vi "Initialize.vi"(0 "VISA resource name":refnum<visa-resource-name>, 7 "Serial Configuration":T1={"Baud Rate (19200)"=19200, "Parity (0: None)"=0, "Break Length (0)"=20} {"Break Length (0)" items=["0"=10, "1.5"=15, "2.0"=20]; "Parity (0: None)" items=["None", "Odd", "Even"]; "Baud Rate (19200)" items=["1200"=1200, "2400"=2400, "4800"=4800, "9600"=9600, "19200"=19200]}, 11 "error in (no error)":errorcluster) -> (4 "VISA resource name out":refnum<visa-resource-name>, 15 "error out":errorcluster {"code" format="%x"})   [LabVIEW 2010, in "Eurotherm 32xx Series.lvlib"]
doc: "This VI passes the addressing information in the instrument decriptor to the Instr Open VI and returns the instrument ID. You must run this VI before using any of the instrument driver VIs for this instrument.\n\nNotes:\n\n(1) This instrument driver supports serial communication. If problems are encountered when using serial communication, it is recommended to try using baud rates less than 19,200 and hardware handshaking. \n\n(2) If you do wish to use the serial interface, set the serial settings on the instrument to be the same as the serial settings on the block diagram and in Measurement & Automation Explorer."
uses:
  <instrlib>/Eurotherm 32xx Series/Eurotherm 32xx Series.lvlib
panel:
  # "(c) 2010 <Invensys Eurotherm>.  ALL RIGHTS RESERVED."
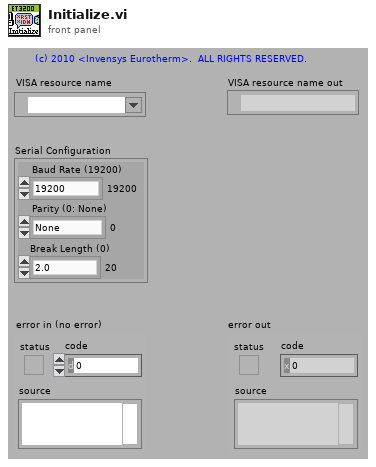
[diagram p1: front panel]
types:
  T1 = cluster{"Baud Rate (19200)":u32, "Parity (0: None)":u16, "Break Length (0)":u16}
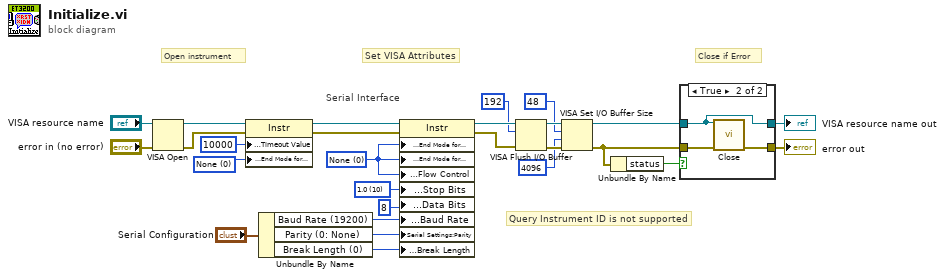
[diagram p0: block diagram]
diagram:
  w5 = u16 10 items=["1.0"=10, "1.5"=15, "2.0"=20] ("Serial Settings:Serial Stop Bits")
  w6 = u16 0 items=["None", "LastBit", "TermChar"] ("Serial Settings:Serial End Mode for Reads")
  w17 = u16 0 items=["None", "LastBit", "TermChar"] ("Serial Settings:Serial End Mode for Reads")
  # "Serial Interface"
  # "Set VISA Attributes"
  # "Close if Error"
  # "Query Instrument ID is not supported"
  # "Open instrument"
  n1 = VISA Open(error in (no error)="error in (no error)", VISA resource name="VISA resource name") -> (VISA resource name=w16:refnum<visa-resource-name>, error out=w15:errorcluster)  [unwired: 3 in]
  n2 = property class="Instr"(reference=w16, error in=w15, "General Settings:Timeout Value"=u32 10000, "Serial Settings:End Mode for Reads"=w17) -> (reference out=w20:refnum<visa-resource-name>, error out=w19:errorcluster)
  n3 = Unbundle By Name("Serial Configuration") -> ("Baud Rate (19200)"=w3:u32, "Parity (0: None)"=w2:u16, "Break Length (0)"=w1:u16)
  n4 = property class="Instr"(reference=w20, error in=w19, "Serial Settings:End Mode for Reads"=w6, "Serial Settings:End Mode for Writes"=w6, "Serial Settings:Flow Control"=w6, "Serial Settings:Stop Bits"=w5, "Serial Settings:Data Bits"=u16 8 ("Serial Settings:Serial Data Bits"), "Serial Settings:Baud Rate"=w3, "Serial Settings:Parity"=w2, "Serial Settings:Break Length"=w1) -> (reference out=w11:refnum<visa-resource-name>, error out=w13:errorcluster)
  n5 = VISA Flush I/O Buffer(VISA resource name=w11, mask (16)=u16 192, error in (no error)=w13) -> (VISA resource name out=w14:refnum<visa-resource-name>, error out=w12:errorcluster)
  n6 = VISA Set I/O Buffer Size(VISA resource name=w14, mask (16)=u16 48, size (4096)=u32 4096 ("size (0)"), error in (no error)=w12) -> (VISA resource name out=w22:refnum<visa-resource-name>, error out=w21:errorcluster)
  n7 = Unbundle By Name(w21) -> ("status"=w18:bool)
  n8 = case shown="True" w18 {
    tunnel: w22 -> [w29 w31]
    tunnel: [w29 w31] -> w27
    tunnel: [w28 w32] -> w26
    tunnel: w21 -> [w28 w30]
    frame False {
    }
    frame True {
      n9 = call <instrlib>:"Close.vi"("VISA resource name"=w31, "error in (no error)"=w30) -> ("error out"=w32:errorcluster)  [unwired: 13 in]
    }
  }
  "VISA resource name out" <- w27
  "error out" <- w26
